vi "simulate.vi"(8 "error in (no error)":errorcluster, 9 "Function":i32, 10 "Address":i32, 11 "Mockbus in":refnum<class "Mockbus.lvclass">) -> (0 "error out":errorcluster, 3 "Mockbus out":refnum<class "Mockbus.lvclass">)   [LabVIEW 2015, in "RTMockbus.lvlib" / "Mockbus.lvclass"]
uses:
  Mockbus.lvclass
  Mockbus.lvclass/Mockbus.ctl
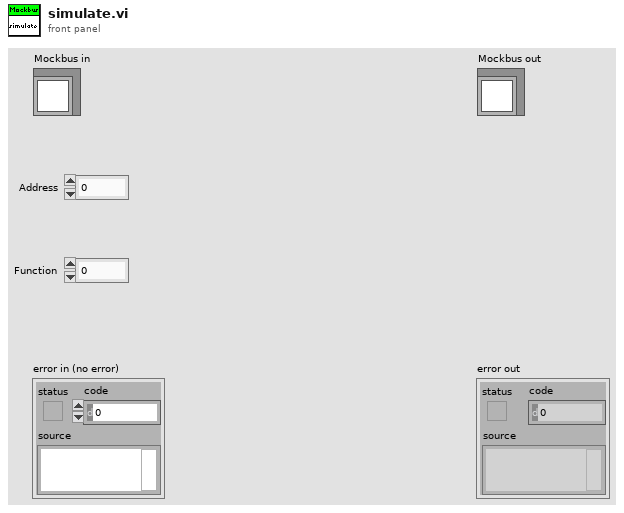
[diagram p1: front panel]
types:
  T1 = typedef "RTModbus.lvlib/Frame.ctl" = cluster{"Data":u8[], "WaitForTrigger":bool, "WaitForRx":u16, "TriggerIRQ":bool, "DelayTicks":u16, "DelayMicroseconds":u16, "DelayMilliseconds":u16}
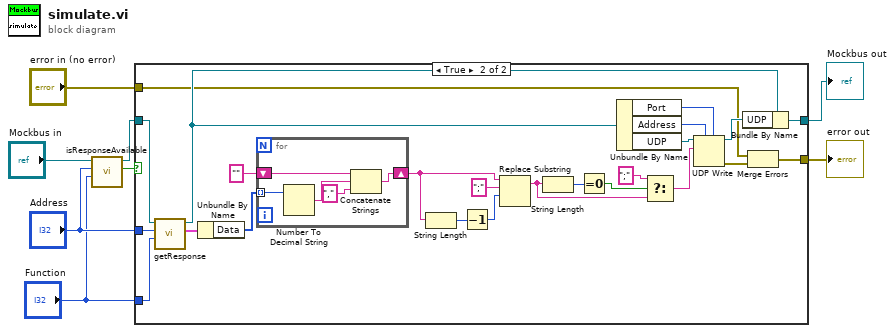
[diagram p0: block diagram]
diagram:
  n1 = call "isResponseAvailable.vi"("Function"="Function", "Address"="Address", "Mockbus in"="Mockbus in") -> ("Available"=w2:bool, "Mockbus out"=w5:refnum<class "Mockbus.lvclass">)  [unwired: 6 in, 1 out]
  n2 = case shown="True" w2 {
    tunnel: [w10 w30] -> w8
    tunnel: [w9 w27] -> w7
    tunnel: w5 -> [w10 w14]
    tunnel: "Address" -> [_ w13]
    tunnel: "Function" -> [_ w12]
    tunnel: "error in (no error)" -> [w9 w11]
    frame False {
    }
    frame True {
      n3 = call "getResponse.vi"("Function"=w12, "Address"=w13, "Mockbus in"=w14) -> ("Frame"=w26:T1, "Mockbus out"=w31:refnum<class "Mockbus.lvclass">)  [unwired: 6 in, 1 out]
      n4 = Unbundle By Name(w26) -> ("Data"=w25:u8[])
      n5 = for {
        tunnel: w25 -> [w38] mode=indexing
        shift-right: [w37] -> w16
        shift-left: "" -> [w36]
        n6 = Number To Decimal String(number=w38) -> (decimal integer string=w39:string)  [unwired: 1 in]
        n7 = Concatenate Strings(w36, w39, "," ("string")) -> (w37:string)
      }
      n8 = String Length(string=w16) -> (length=w18:i32)
      n9 = Decrement(x=w18) -> (x-1=w17:i32)
      n10 = Replace Substring(3:w17, 4:";" ("substring (\"\")"), 5:w16) -> (1:w22:string)  [unwired: 1 in, 1 out]
      n11 = String Length(string=w22) -> (length=w20:i32)
      n12 = Equal To 0?(x=w20) -> (x = 0?=w21:bool)
      n13 = Unbundle By Name(w31) -> ("Port"=w32:u16, "Address"=w33:u32, "UDP"=w34:refnum<k16>)
      n14 = Select(t=";", s=w21, f=w22) -> (s? t:f=w15:string)
      n15 = UDP Write(address=w33, port or service name=w32, connection ID=w34, data in=w15) -> (error out=w28:errorcluster, 3:w29:refnum<k16>)  [unwired: 2 in]
      n16 = Bundle By Name(cluster=w31, "UDP"=w29) -> (w30:refnum<class "Mockbus.lvclass">)
      n17 = Merge Errors(w11, w28) -> (w27:errorcluster)
    }
  }
  "error out" <- w7
  "Mockbus out" <- w8
